vi "PH_Beckhoff_PP_PU.calc PSU State.vi"(1 "GUI Refs: HV on indicator, sum fault and end of charge":refnum<vi>[](array[refnum]), 2 "# in Data: HV on indicator, sum fault and end of charge":i32[](array[numeric]), 3 "Digital Inputs":T1, 5 "error in":errorcluster) -> (17 "PSU Status":T2 items=["no info", "off/false/out", "on/true/in", "Failure", "Alarm", "Status 1", "Status 2", "Status 3"], 19 "error out":errorcluster)   [LabVIEW 2014, in "PH_Beckhoff_PP_PU.lvlib"]
uses:
  PH_Beckhoff_PP_PU.lvlib
  PH_StatusHandler/PH_StatusHandler.Status.ctl
  PH_Beckhoff/PH_Beckhoff.Digital Inputs.ctl
  PH_StatusHandler/PH_StatusHandler.lvlib
  PH_Beckhoff/PH_Beckhoff.lvlib
  PH_Common/PH_Common.lvlib
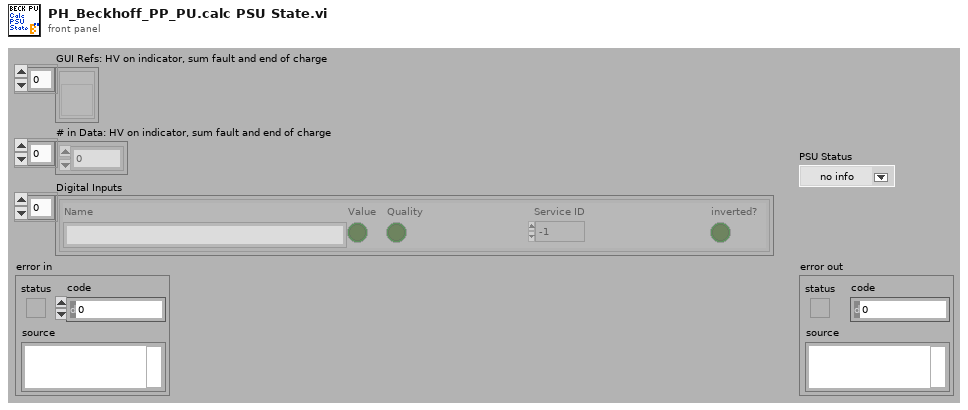
[diagram p1: front panel]
types:
  T1 = typedef "PH_Beckhoff.lvlib/PH_Beckhoff.Digital Inputs.ctl" = cluster{"Name":string, "Value":bool, "Quality":bool, "Service ID":i32, "inverted?":bool}[]
  T2 = typedef "PH_StatusHandler.lvlib/PH_StatusHandler.Status.ctl" = i16
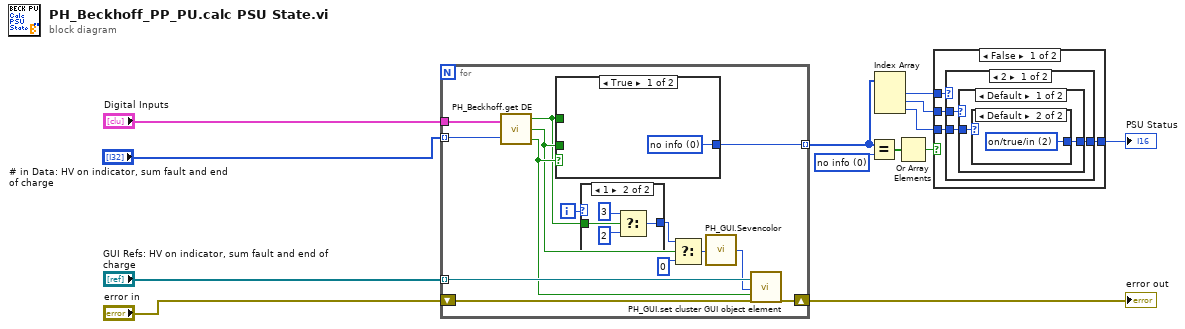
[diagram p0: block diagram]
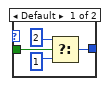
[diagram p2: hidden frame]
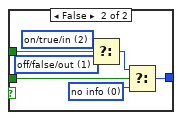
[diagram p3: hidden frame]
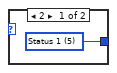
[diagram p4: hidden frame]
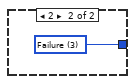
[diagram p5: hidden frame]
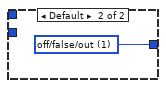
[diagram p6: hidden frame]
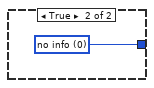
[diagram p7: hidden frame]
diagram:
  w7 = T2 0 items=["no info", "off/false/out", "on/true/in", "Failure", "Alarm", "Status 1", "Status 2", "Status 3"] ("EOC State")
  n1 = for {
    tunnel: [w27] -> w6 mode=indexing
    tunnel: "Digital Inputs" -> [w26]
    tunnel: "# in Data: HV on indicator, sum fault and end of charge" -> [w25] mode=indexing
    shift-right: [w24] -> w3
    shift-left: "error in" -> [w23]
    tunnel: "GUI Refs: HV on indicator, sum fault and end of charge" -> [w22] mode=indexing
    i -> [w16]
    n2 = call "PH_Beckhoff.get DE.vi"("Digital Values"=w26, "index of element"=w25) -> ("Value"=w17:bool, "Quality"=w18:bool, "Tag not found"=w19:bool)
    n3 = case shown="True" w19 {
      tunnel: [w36 w43] -> w27
      tunnel: w18 -> [_ w38]
      tunnel: w17 -> [_ w37]
      frame True {
        w36 = T2 0 items=["no info", "off/false/out", "on/true/in", "Failure", "Alarm", "Status 1", "Status 2", "Status 3"] ("HV On State")
      }
      frame False {
        w39 = T2 1 items=["no info", "off/false/out", "on/true/in", "Failure", "Alarm", "Status 1", "Status 2", "Status 3"] ("HV On State")
        w40 = T2 2 items=["no info", "off/false/out", "on/true/in", "Failure", "Alarm", "Status 1", "Status 2", "Status 3"] ("HV On State")
        w42 = T2 0 items=["no info", "off/false/out", "on/true/in", "Failure", "Alarm", "Status 1", "Status 2", "Status 3"] ("HV On State")
        n4 = Select(t=w40, s=w37, f=w39) -> (s? t:f=w41:T2)
        n5 = Select(t=w41, s=w38, f=w42) -> (s? t:f=w43:T2)
      }
    }
    n6 = case shown="1" w16 {
      tunnel: w17 -> [w31 w35]
      tunnel: [w28 w32] -> w20
      frame Default {
        n7 = Select(t=2 ("State"), s=w31, f=1 ("State")) -> (s? t:f=w28:i32)
      }
      frame 1 {
        n8 = Select(t=3 ("State"), s=w35, f=2 ("State")) -> (s? t:f=w32:i32)
      }
    }
    n9 = Select(t=w20, s=w18, f=0 ("State")) -> (s? t:f=w21:i32)
    n10 = call "PH_GUI.Sevencolor.vi"("State"=w21) -> ("Color Box"=w14:u32)
    n11 = call "PH_GUI.set cluster GUI object element.vi"("Ctl Refnum"=w22, "Value"=w14, "Blinking? (false)"=w19, "error in"=w23) -> ("error out"=w24:errorcluster)  [unwired: 15 in]
  }
  "error out" <- w3
  n12 = Equal?(x=w6, y=w7) -> (x = y?=w8:bool[])
  n13 = Index Array(array=w6) -> (element #1=w10:T2, element #2=w11:T2, element #3=w12:T2)  [unwired: 3 in]
  n14 = Or Array Elements(Boolean array=w8) -> (logical OR=w9:bool)
  n15 = case shown="False" w9 {
    tunnel: [w46 w57] -> w13
    tunnel: w12 -> [w44 _]
    tunnel: w11 -> [w45 _]
    tunnel: w10 -> [w47 _]
    frame False {
      n16 = case shown="2" w47 {
        tunnel: [w49 w56] -> w46
        tunnel: w45 -> [w50 _]
        tunnel: w44 -> [w48 _]
        frame 2 {
          n17 = case shown="Default" w50 {
            tunnel: [w51 w55] -> w49
            tunnel: w48 -> [w52 _]
            frame Default {
              n18 = case shown="Default" w52 {
                tunnel: [w53 w54] -> w51
                frame 2 {
                  w53 = T2 5 items=["no info", "off/false/out", "on/true/in", "Failure", "Alarm", "Status 1", "Status 2", "Status 3"] ("Device Status")
                }
                frame Default {
                  w54 = T2 2 items=["no info", "off/false/out", "on/true/in", "Failure", "Alarm", "Status 1", "Status 2", "Status 3"] ("Device Status")
                }
              }
            }
            frame 2 {
              w55 = T2 3 items=["no info", "off/false/out", "on/true/in", "Failure", "Alarm", "Status 1", "Status 2", "Status 3"] ("Device Status")
            }
          }
        }
        frame Default {
          w56 = T2 1 items=["no info", "off/false/out", "on/true/in", "Failure", "Alarm", "Status 1", "Status 2", "Status 3"] ("Device Status")
        }
      }
    }
    frame True {
      w57 = T2 0 items=["no info", "off/false/out", "on/true/in", "Failure", "Alarm", "Status 1", "Status 2", "Status 3"] ("Device Status")
    }
  }
  "PSU Status" <- w13
